vi "111_config.vi"() -> ()   [LabVIEW 2019]
panel:
  out "XY图":cluster{"X":dbl, "Y":dbl}[](graph)
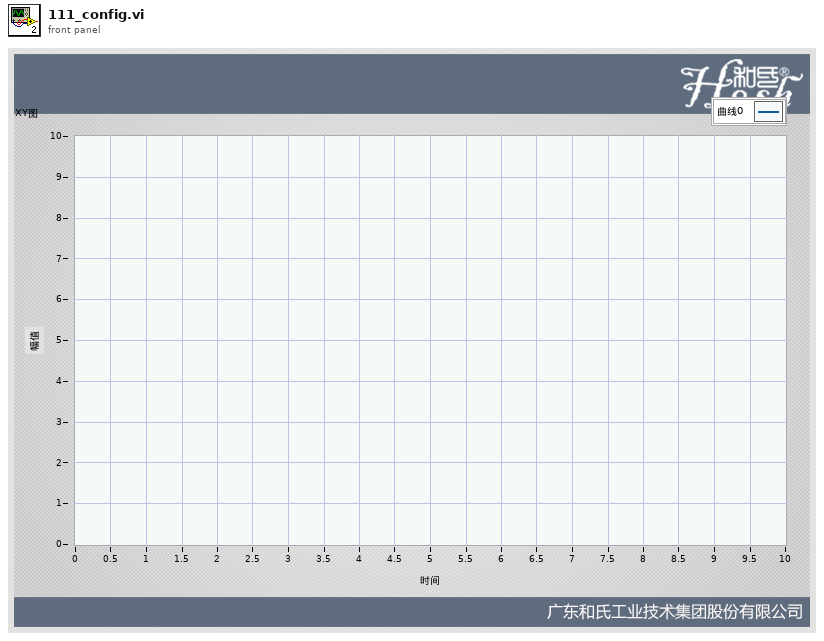
[diagram p1: front panel]
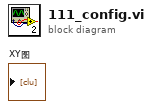
[diagram p0: block diagram]
diagram:
